vi "DRIVE_STRAIGHT_TARGET.vi"(10 "argv":string[](array[string]), 11 "args":u8) -> ()   [LabVIEW 2015]
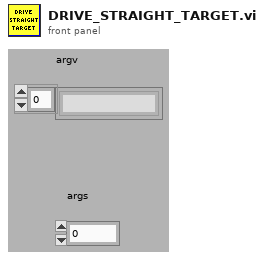
[diagram p1: front panel]
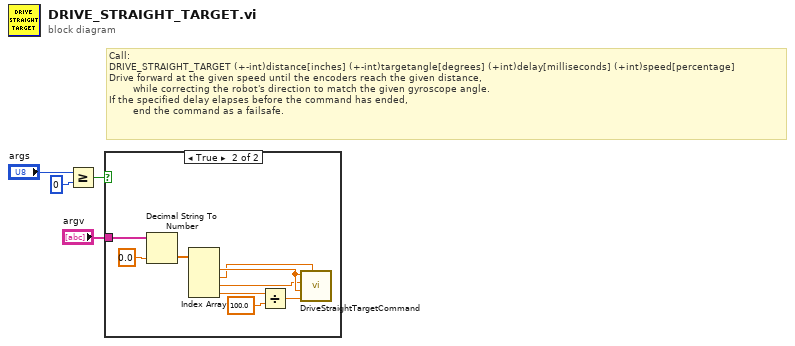
[diagram p0: block diagram]
diagram:
  # "Call:\nDRIVE_STRAIGHT_TARGET (+-int)distance[inches] (+-int)targetangle[degrees] (+int)delay[milliseconds] (+int)speed[percentage]\nDrive forward at the given speed until the encoders reach the given distance,\n        while correcting the robot's direction to match the given gyroscope angle.\nIf the specified delay elapses before the command has ended,\n        end the command as a failsafe."
  n1 = Greater Or Equal?(x="args", y=u8 0) -> (x >= y?=w4:bool)
  n2 = case shown="True" w4 {
    tunnel: "argv" -> [_ w13]
    frame False {
    }
    frame True {
      n3 = Decimal String To Number(string=w13, default (0L)=0.0 ("default (0 I32)")) -> (number=w11:dbl[])  [unwired: 2 out]
      n4 = Index Array(array=w11) -> (element #1=w10:dbl, element #2=w9:dbl, element #3=w8:dbl, element #4=w6:dbl)  [unwired: 4 in]
      n5 = Divide(x=w6, y=100.0) -> (x/y=w7:dbl)
      n6 = call "DriveStraightTargetCommand.vi"("Navx Target"=w9, "speed"=w7, "Fwd Bwd"=w10, "Delay ms"=w8, "distance"=w10) -> ()  [unwired: 7 in]
    }
  }
